vi "rs3 get frame data2.vi"(8 "error in (no error)":errorcluster, 9 "size":cluster{"width":u32, "height":u32}, 10 "stream type":u16(ring) items=["depth", "color", "inf 1", "inf 2"], 11 "device in":u64) -> (0 "error out":errorcluster, 1 "2D Color Output":u32[][](array[numeric]), 2 "2D Depth Output":u16[][](array[numeric]), 3 "device out":u64)   [LabVIEW 2017, in "libRealSense3.lvlib"]
doc: "With a FRAME handle as input, this will return a pointer to the actual image data. \nUse the different MEMCOPY VIs to copy the data into LabVIEW."
uses:
  <vilib>/addons/RealSense/libRealSense3.lvlib
  <vilib>/addons/RealSense/realsense-d.dll
panel:
  # "RS3 Get Frame Data 2"
  # "(C) Intel Corp. 2017,  AGJ"
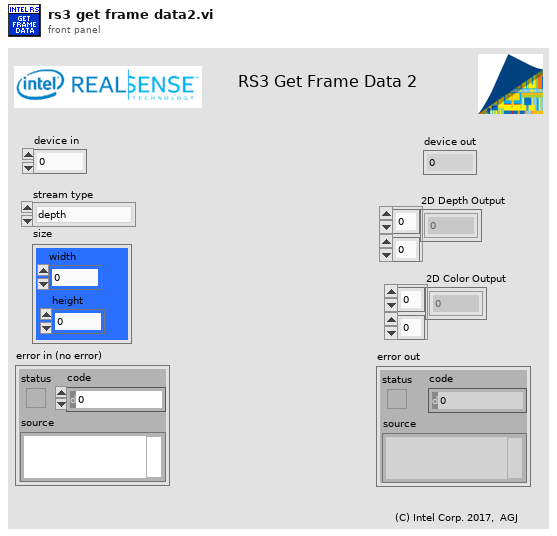
[diagram p1: front panel]
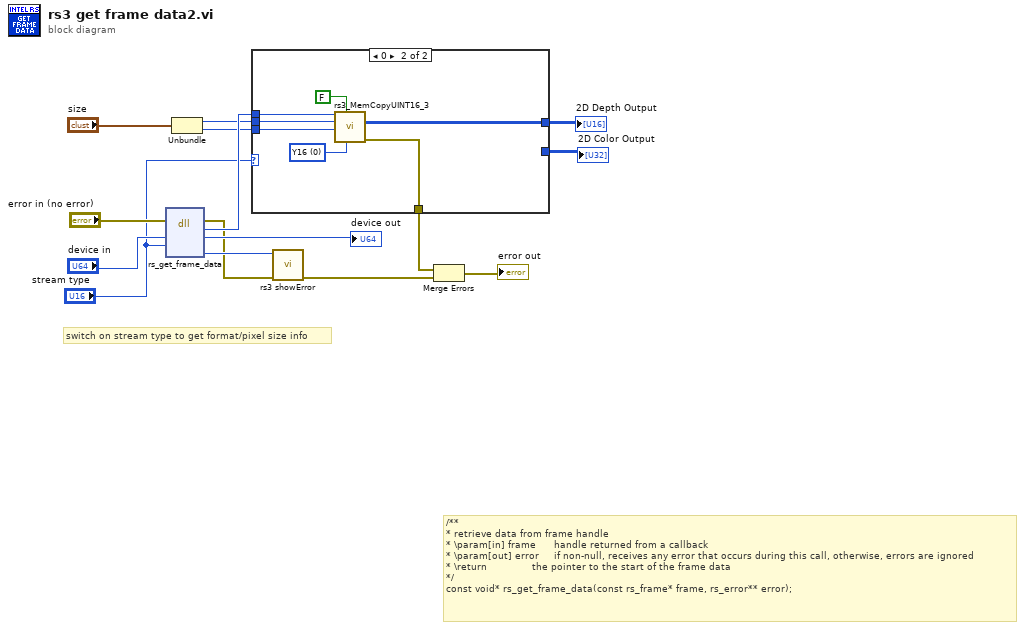
[diagram p0: block diagram]
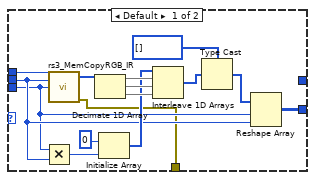
[diagram p2: hidden frame]
diagram:
  # "switch on stream type to get format/pixel size info"
  # "/**\n* retrieve data from frame handle\n* \\param[in] frame      handle returned from a callback\n* \\param[out] error     if non-null, receives any error that occurs during this call, otherwise, errors are ignored\n* \\return               the pointer to the start of the frame data\n*/\nconst void* rs_get_frame_data(const rs_frame* frame, rs_error** error);"
  n1 = dll-call lib="C:/Program Files (x86)/National Instruments/LabVIEW 2017/vi.lib/addons/RealSense/realsense-d.dll" fn="rs_get_frame_data"(error in="error in (no error)", "device"="device in", "streamType"="stream type") -> (error out=w10:errorcluster, "return type"=w12:u64, "device"=→"device out":u64, "error"=w11:u64)  [unwired: 4 in, 1 out]
  n2 = Unbundle("size") -> ("width"=w6:u32, "height"=w5:u32)
  n3 = case shown="0" "stream type" {
    tunnel: w12 -> [w30 w37]
    tunnel: [_ w35] -> w8
    tunnel: w6 -> [w21 w33]
    tunnel: w5 -> [w20 w32]
    tunnel: [w24 _] -> w4
    tunnel: [w16 w31] -> w1
    frame Default {
      n4 = Multiply(x=w20, y=w21) -> (x*y=w23:u32)
      n5 = call <vilib>:"rs3_MemCopyRGB_IR.vi"("Zimage pointer"=w30, "RGB  X, width"=w21, "RGB Y, height"=w20) -> ("Output Array"=w29:u8[], "error out"=w16:errorcluster)  [unwired: 11 in]
      n6 = Decimate 1D Array(w29) -> (w28:u8[], w27:u8[], w26:u8[])
      n7 = Initialize Array(u8 0, w23) -> (w22:u8[])
      n8 = Interleave 1D Arrays(w22, w28, w27, w26) -> (w19:u8[])
      n9 = Type Cast(type=u32[] [], x=w19) -> (*(type *) &x=w18:u32[])
      n10 = Reshape Array(w18, w20, w21) -> (w24:u32[][])
    }
    frame 0 {
      w36 = u16 0 items=["Y16", "Y8"] ("Image format")
      n11 = call <vilib>:"rs3_MemCopyUINT16_3.vi"("Image format"=w36, "Transpose"=FALSE, "Height"=w32, "Width"=w33, "Zimage pointer"=w37) -> ("error out"=w31:errorcluster, "2D Array Output"=w35:u16[][])  [unwired: 5 in]
    }
  }
  "2D Depth Output" <- w8
  "2D Color Output" <- w4
  n12 = call <vilib>:"rs3 showError.vi"("error in (no error)"=w10, "error"=w11) -> ("error out"=w2:errorcluster)  [unwired: 5 in, 4 out]
  n13 = Merge Errors(w1, w2) -> (→"error out":errorcluster)
